vi "Launch View.vi"(8 "error in (no error)":errorcluster, 9 "Actor":refnum<class "Actor.lvclass">, 10 "Name":string, 11 "MVVM Abstruct Model in":refnum<class "MVVM Abstruct Model.lvclass">) -> (0 "error out":errorcluster, 3 "MVVM Abstruct Model out":refnum<class "MVVM Abstruct Model.lvclass">)   [LabVIEW 2020, in "MMVVM Framework.lvlib" / "MVVM Abstruct Model.lvlib" / "MVVM Abstruct Model.lvclass"]
uses:
  MVVM Abstruct Model.lvclass
  <vilib>/ActorFramework/Actor/Actor.lvclass
  C:/Program Files (x86)/National Instruments/LabVIEW 2020/vi.lib/ActorFramework/Actor/Actor.lvclass
  <vilib>/ActorFramework/Message/Message.lvclass
  MVVM Abstruct Model.lvclass/MVVM Abstruct Model.ctl
  <vilib>/ActorFramework/Actor/Actor.lvclass/Actor.ctl
  <vilib>/ActorFramework/Message Enqueuer/Message Enqueuer.lvclass/Message Enqueuer.ctl
  Enqueues Data/Enqueues Data.lvclass
  Enqueues Data/Enqueues Data.lvclass/Enqueues Data.ctl
  MVVM Abstruct Controller/MVVM Abstruct Controller Messages/Add & Register Views Msg/Add & Register Views Msg.lvclass/Add & Register Views Msg.ctl
  Enqueues Data/Accessors/Write ActorMap.vi
  MVVM Abstruct Controller/MVVM Abstruct Controller Messages/Add & Register Views Msg/Add & Register Views Msg.lvclass
  C:/Program Files (x86)/National Instruments/LabVIEW 2020/vi.lib/ActorFramework/Message/Message.lvclass
  <vilib>/ActorFramework/Message Priority Queue/Priority Enqueue.vi
  ActorMap/ActorMap.lvclass
  <vilib>/ActorFramework/Message Enqueuer/Message Enqueuer.lvclass
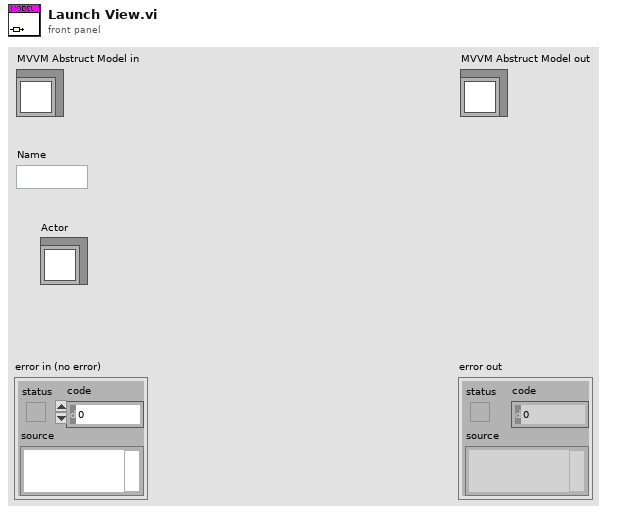
[diagram p1: front panel]
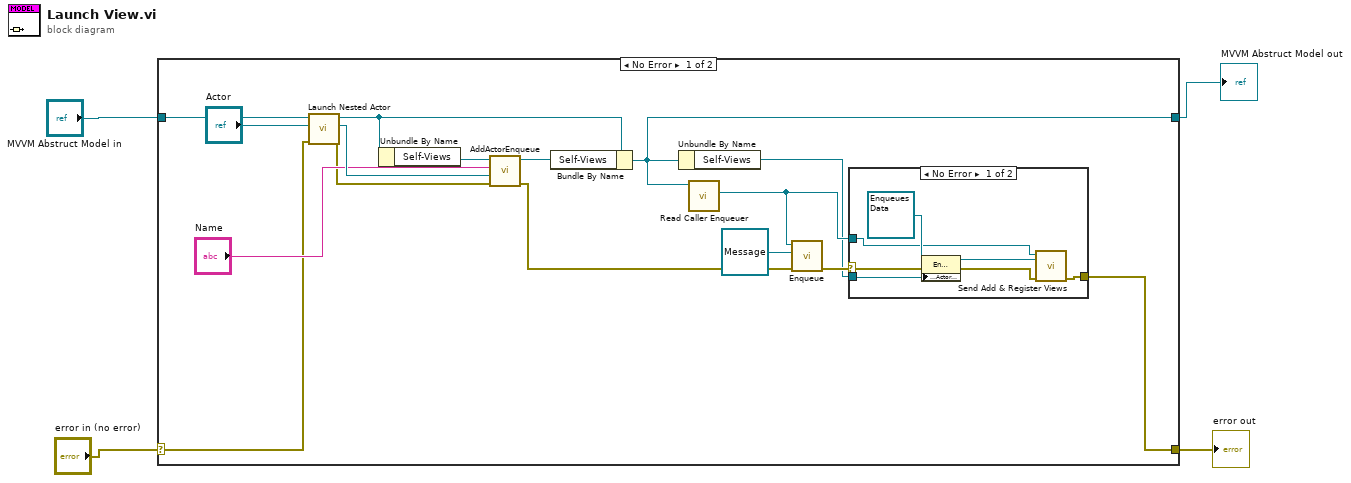
[diagram p0: block diagram]
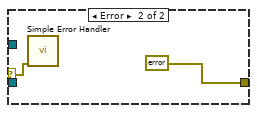
[diagram p2: hidden frame]
diagram:
  n1 = case shown="No Error" "error in (no error)" {
    selector: "error in (no error)" -> [w6 w31]
    tunnel: [w7 w31] -> w1
    tunnel: [w8 w30] -> w2
    tunnel: "MVVM Abstruct Model in" -> [w20 w30]
    frame No Error {
      n2 = call <vilib>:"Launch Nested Actor.vi"("error in (no error)"=w6, "Nested Actor"="Actor", "Caller Actor in"=w20) -> ("error out"=w5:errorcluster, "Nested Actor's Enqueuer"=w15:refnum<class "Message Enqueuer.lvclass">, "Caller Actor out"=w18:refnum<class "MVVM Abstruct Model.lvclass">)  [unwired: 6 in]
      n3 = Unbundle By Name(w18) -> ("Self-Views"=w17:refnum<class "ActorMap.lvclass">)
      n4 = call "AddActorEnqueue.vi"("error in (no error)"=w5, "Actor's Enqueuer"=w15, "name"="Name", "ActorMap in"=w17) -> ("error out"=w9:errorcluster, "ActorMap out"=w16:refnum<class "ActorMap.lvclass">)  [unwired: 6 in]
      n5 = Bundle By Name(cluster=w18, "Self-Views"=w16) -> (w8:refnum<class "MVVM Abstruct Model.lvclass">)
      n6 = Unbundle By Name(w8) -> ("Self-Views"=w10:refnum<class "ActorMap.lvclass">)
      n7 = call <vilib>:"Read Caller Enqueuer.vi"("Actor"=w8) -> ("Caller Enqueuer"=w11:refnum<class "Message Enqueuer.lvclass">)  [unwired: 10 in]
      n8 = call <vilib>:"Enqueue.vi"("error in (no error)"=w9, "Message"=refnum<class "Message.lvclass"> refnum, "Message Enqueuer in"=w11) -> ("error out"=w12:errorcluster)  [unwired: 7 in, 1 out]
      n9 = case shown="No Error" w12 {
        selector: w12 -> [w25 w29]
        tunnel: [w21 errorcluster {"status"=FALSE, "code"=0, "source"=""} ("error out")] -> w7
        tunnel: w11 -> [w24 _]
        tunnel: w10 -> [w26 _]
        frame No Error {
          n10 = property class="Enqueues Data.lvclass"(reference=refnum<class "Enqueues Data.lvclass"> refnum ("View"), error in=w25, "Accessors:ActorMap"=w26) -> (reference out=w23:refnum<class "Enqueues Data.lvclass">, error out=w22:errorcluster)
          n11 = call "Send Add & Register Views.vi"("error in (no error)"=w22, "View"=w23, "Message Enqueuer"=w24) -> ("error out"=w21:errorcluster)  [unwired: 7 in, 1 out]
        }
        frame Error {
          n12 = call <vilib>:"Simple Error Handler.vi"("error in (no error)"=w29) -> ()  [unwired: 4 in, 5 out]
        }
      }
    }
    frame Error {
    }
  }
  "error out" <- w1
  "MVVM Abstruct Model out" <- w2
